vi "Write Vertical Arrangement.vi"(5 "Vertical Arrangement":T1(ring), 9 "Text in":refnum<class "Text.lvclass">) -> (3 "Text out":refnum<class "Text.lvclass">)   [LabVIEW 2014, in "Text.lvclass"]
uses:
  Text.lvclass
  Text.lvclass/Text.ctl
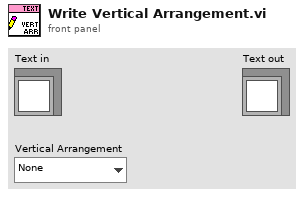
[diagram p1: front panel]
types:
  T1 = enum16{"None", "Stacked", "Clockwise", "Counterclockwise"}
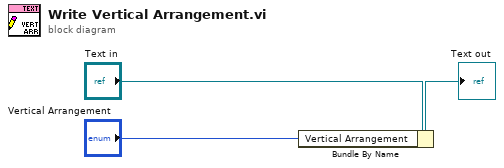
[diagram p0: block diagram]
diagram:
  n1 = Bundle By Name(cluster="Text in", "Vertical Arrangement"="Vertical Arrangement") -> (→"Text out":refnum<class "Text.lvclass">)
